vi "Update Progress Window.vi"(7 "stop (F)":bool, 8 "error in (no error)":errorcluster, 9 "progress (0)":dbl, 10 "message (\"\")":string, 11 "progress queue in":refnum<queue>) -> (0 "error out":errorcluster, 3 "progress queue out":refnum<queue>)   [LabVIEW 2020, in "DSF System Explorer.lvlib"]
uses:
  DSF System Explorer.lvlib
  progress window data.ctl
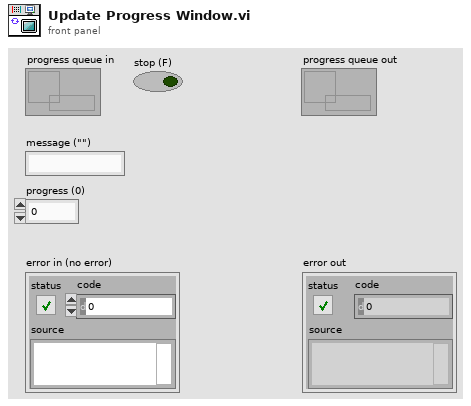
[diagram p1: front panel]
types:
  T1 = typedef "DSF System Explorer.lvlib/progress window data.ctl" = cluster{"stop":bool, "message":string, "progress":dbl}
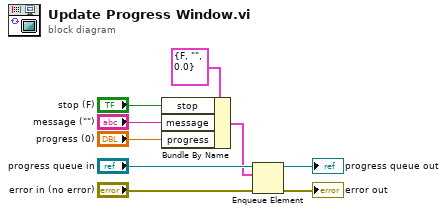
[diagram p0: block diagram]
diagram:
  n1 = Bundle By Name(cluster=T1 {"stop"=FALSE, "message"="", "progress"=0.0} ("element"), "stop"="stop (F)", "message"="message (\"\")", "progress"="progress (0)") -> (w1:T1)
  n2 = Enqueue Element(queue="progress queue in", element=w1, error in (no error)="error in (no error)") -> (queue out=→"progress queue out":refnum<queue>, error out=→"error out":errorcluster)  [unwired: 1 in, 1 out]
